vi "test Action Update Ramp Rate-errorCase.vi"() -> ()   [LabVIEW 2018, in "AllComponentTestes.lvclass"]
uses:
  AllComponentTestes.lvclass
  C:/Program Files/National Instruments/LabVIEW 2018/vi.lib/addons/_JKI Toolkits/VI Tester/TestCase.llb/TestCase.lvclass
  <vilib>/addons/_JKI Toolkits/VI Tester/TestCase.llb/TestCase.lvclass
  Libraries/Thermal Chamber Controller_DQMH/Thermal Chamber Controller_DQMH.lvlib
panel:
  out "TestCase out":refnum<class "TestCase.lvclass">
  in  "TestCase in":refnum<class "AllComponentTestes.lvclass">
  out "error out":errorcluster
  in  "error in (no error)":errorcluster
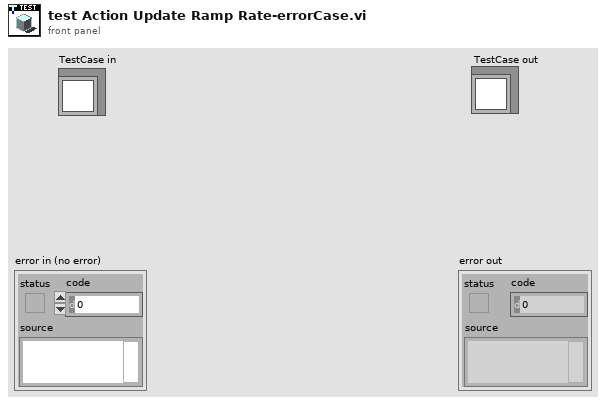
[diagram p1: front panel]
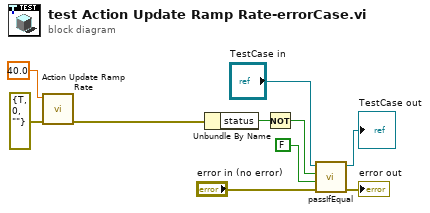
[diagram p0: block diagram]
diagram:
  n1 = call "Action Update Ramp Rate.vi"("error in (no error)"=errorcluster {"status"=TRUE, "code"=0, "source"=""}, "Temperature Ramp Rate"=40.0 ("Temperature Set Point")) -> ("error out"=w4:errorcluster)  [unwired: 9 in]
  n2 = Unbundle By Name(w4) -> ("status"=w5:bool)
  n3 = Not(x=w5) -> (.not. x?=w3:bool)
  n4 = call-dynamic "passIfEqual.vi"("error in (no error)"="error in (no error)", "y"=FALSE, "x"=w3, "TestCase in"="TestCase in") -> ("error out"=→"error out":errorcluster, "TestCase out"=→"TestCase out":refnum<class "AllComponentTestes.lvclass">)  [unwired: 6 in]
